vi "get full tag list.vi"(11 "engine configuration in":refnum<class "engine configuration.lvclass">) -> (2 "tag list":refnum<class "tag descriptor.lvclass">[](array[class]), 3 "engine configuration out":refnum<class "engine configuration.lvclass">)   [LabVIEW 2014, in "engine configuration.lvclass"]
doc: "Returns the full list of Tags that the engine has been configured to create."
uses:
  engine configuration.lvclass
  <vilib>/NI/Tag Bus/tag/tag descriptor.lvclass
  engine configuration.lvclass/engine configuration.ctl
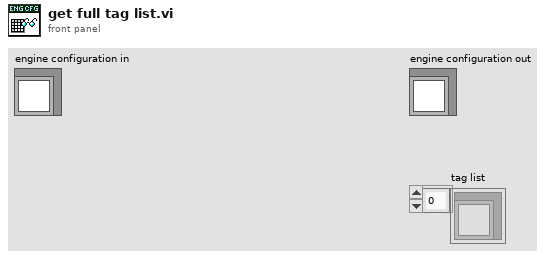
[diagram p1: front panel]
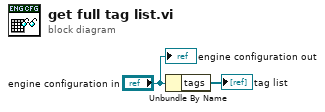
[diagram p0: block diagram]
diagram:
  n1 = Unbundle By Name("engine configuration in") -> ("tags"=→"tag list":refnum<class "tag descriptor.lvclass">[])
  "engine configuration out" <- "engine configuration in"
